vi "23384_Davis_Poku_Amankwa_Amankwa.DavisPoku.MNE1201.6.3_348261_1019197086.vi"() -> ()   [LabVIEW 2018]
panel:
  out "String":string
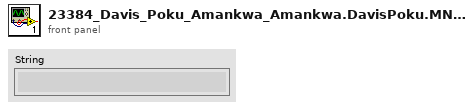
[diagram p1: front panel]
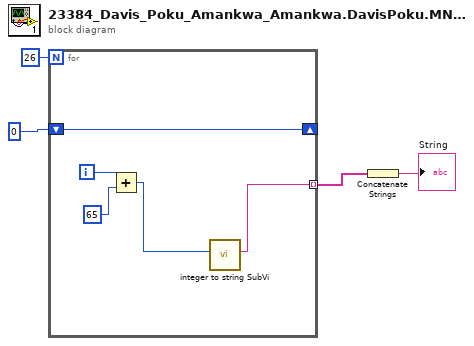
[diagram p0: block diagram]
diagram:
  n1 = for {
    N: 26 -> [_]
    shift-right: [w8] -> _
    shift-left: 0 -> [w8]
    tunnel: [w6] -> w2 mode=indexing
    i -> [w5]
    n2 = Add(x=w5, y=65) -> (x+y=w7:i32)
    n3 = call "integer to string SubVi.vi"("integer input"=w7) -> ("String output"=w6:string)  [unwired: 10 in]
  }
  n4 = Concatenate Strings(w2) -> (→"String":string)
